vi "Configure Sys (To) Input.vi"(4 "Sys Gate Lev (2.5)":dbl=2.5 format="%.4p", 5 "Sys Trig Lev (2.5)":dbl=2.5 format="%.4p", 6 "Sys Gate Mode":T1(ring), 7 "Sys Trig Edge (T: Rising)":bool=TRUE, 8 "error in (no error)":errorcluster, 9 "Sys Gate Logic (T:High)":bool=TRUE, 10 "Sys Ext Mode":T2(ring), 11 "VISA resource name":refnum<visa-resource-name>) -> (0 "error out":errorcluster, 3 "VISA resource name out":refnum<visa-resource-name>)   [LabVIEW 2013, in "Berkeley Nucleonics 500 Series.lvlib"]
doc: "This VI is used to configure the trigger and gate modes of operation of the main system time (To).\n\nThe parameters \"Trigger Level\", \"Gate Polarity\", \"Trigger Edge\" are only updated when operating in the corresponding mode."
uses:
  Berkeley Nucleonics 500 Series.lvlib
panel:
  # "Trigger"
  # "Simultaneous gating and triggering are currently only supported by the 575."
  # "Gate"
  # "The parameters \"Trigger Level\", \"Gate Polarity\", \"Trigger Edge\" are only updated when operating in the corresponding mode."
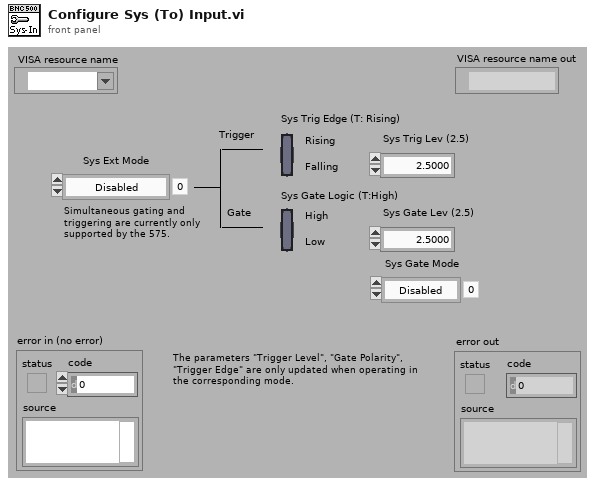
[diagram p1: front panel]
types:
  T1 = enum16{"Disabled", "Pulse Inhibit", "Output Inhibit", "Channel"}
  T2 = enum16{"Disabled", "Triggered", "Gated", "Triggered & Gated"}
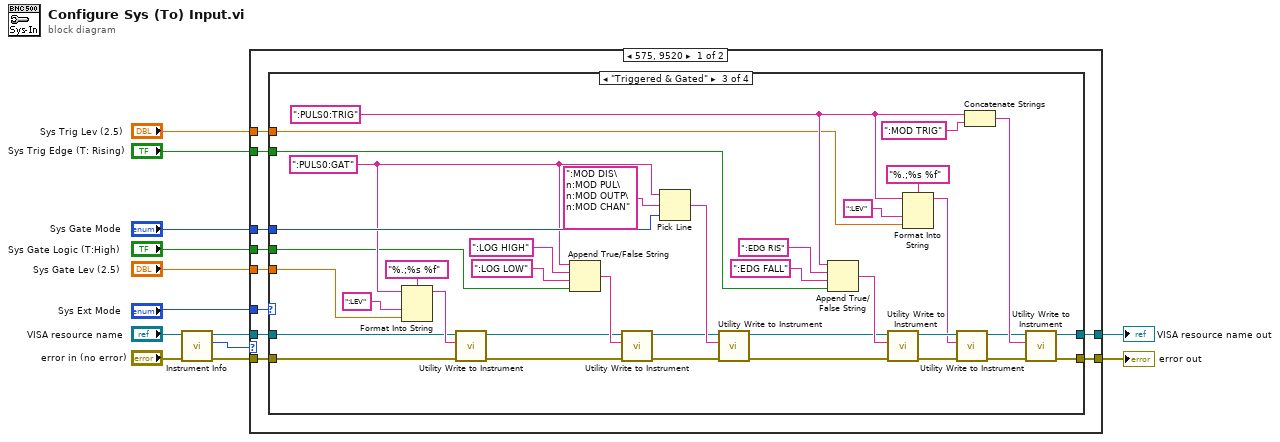
[diagram p0: block diagram]
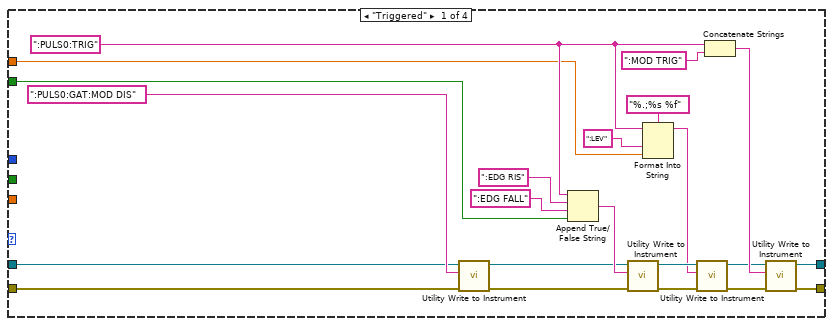
[diagram p2: hidden frame]
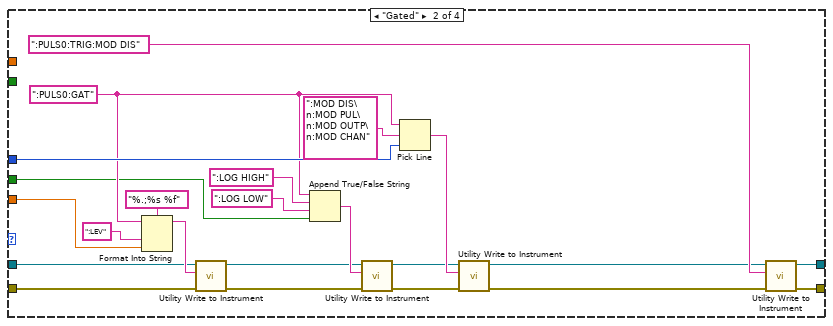
[diagram p3: hidden frame]
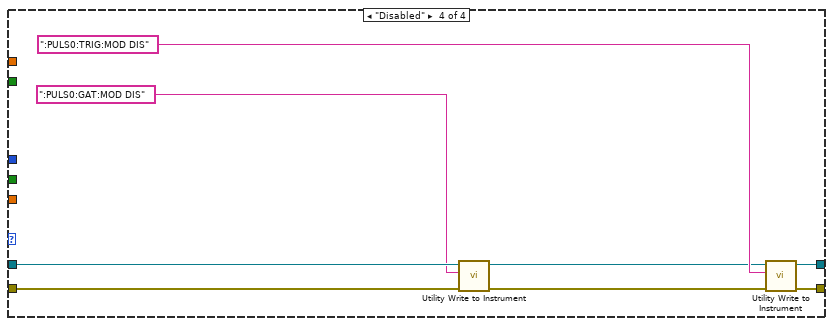
[diagram p4: hidden frame]
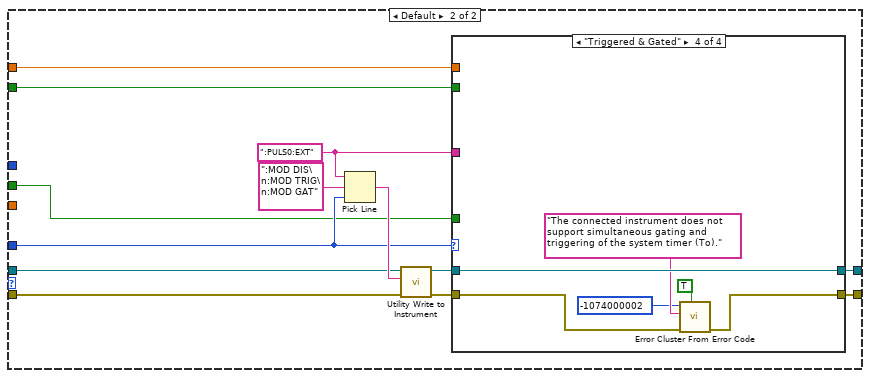
[diagram p5: hidden frame]
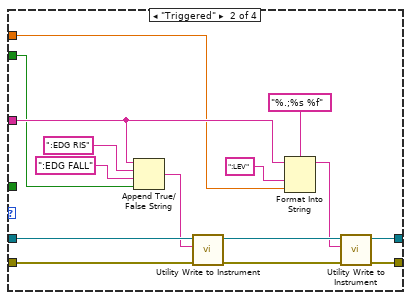
[diagram p7: hidden frame]
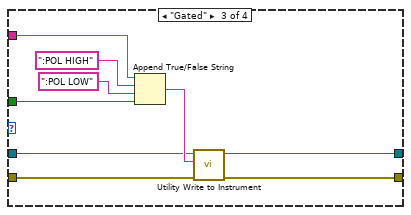
[diagram p8: hidden frame]
diagram:
  n1 = call "Instrument Info.vi"("error in (no error)"="error in (no error)", "VISA resource name"="VISA resource name") -> ("error out"=w8:errorcluster, "Instr Model"=w1:u32, "VISA resource name out"=w7:refnum<visa-resource-name>)  [unwired: 6 in, 1 out]
  n2 = case shown="575, 9520" w1 {
    tunnel: [w23 w121] -> w13
    tunnel: [w22 w120] -> w12
    tunnel: "Sys Ext Mode" -> [w19 w119]
    tunnel: w8 -> [w20 w118]
    tunnel: w7 -> [w21 w117]
    tunnel: "Sys Trig Edge (T: Rising)" -> [w17 w116]
    tunnel: "Sys Trig Lev (2.5)" -> [w18 w115]
    tunnel: "Sys Gate Logic (T:High)" -> [w15 w114]
    tunnel: "Sys Gate Mode" -> [w16 _]
    tunnel: "Sys Gate Lev (2.5)" -> [w14 _]
    frame 575, 9520 {
      n3 = case shown="\"Triggered & Gated\"" w19 {
        tunnel: w21 -> [w25 w54 w76 w108]
        tunnel: w20 -> [w24 w53 w75 w107]
        tunnel: [w41 w65 w99 w112] -> w23
        tunnel: [w42 w66 w100 w113] -> w22
        tunnel: w18 -> [w29 _ w87 _]
        tunnel: w17 -> [w38 _ w96 _]
        tunnel: w16 -> [_ w64 w86 _]
        tunnel: w15 -> [_ w56 w78 _]
        tunnel: w14 -> [_ w55 w77 _]
        frame "Triggered" {
          w30 = ":PULS0:TRIG"
          n4 = call "Utility Write to Instrument.vi"("error in (no error)"=w24, "Write Buffer"=":PULS0:GAT:MOD DIS", "VISA resource name"=w25) -> ("error out"=w27:errorcluster, "VISA resource name out"=w28:refnum<visa-resource-name>)  [unwired: 6 in, 1 out]
          n5 = Append True/False String(1:w38, 2:":EDG FALL", 3:":EDG RIS", 4:w30) -> (0:w43:string)
          n6 = call "Utility Write to Instrument.vi"("error in (no error)"=w27, "Write Buffer"=w43, "VISA resource name"=w28) -> ("error out"=w33:errorcluster, "VISA resource name out"=w32:refnum<visa-resource-name>)  [unwired: 6 in, 1 out]
          n7 = Format Into String(format string="%.;%s %f", initial string=w30, ":LEV", w29) -> (resulting string=w31:string)  [unwired: 1 in, 1 out]
          n8 = call "Utility Write to Instrument.vi"("error in (no error)"=w33, "Write Buffer"=w31, "VISA resource name"=w32) -> ("error out"=w35:errorcluster, "VISA resource name out"=w34:refnum<visa-resource-name>)  [unwired: 6 in, 1 out]
          n9 = Concatenate Strings(w30, ":MOD TRIG") -> (w39:string)
          n10 = call "Utility Write to Instrument.vi"("error in (no error)"=w35, "Write Buffer"=w39, "VISA resource name"=w34) -> ("error out"=w42:errorcluster, "VISA resource name out"=w41:refnum<visa-resource-name>)  [unwired: 6 in, 1 out]
        }
        frame "Gated" {
          w57 = ":PULS0:GAT"
          n11 = Format Into String(format string="%.;%s %f", initial string=w57, ":LEV", w55) -> (resulting string=w63:string)  [unwired: 1 in, 1 out]
          n12 = call "Utility Write to Instrument.vi"("error in (no error)"=w53, "Write Buffer"=w63, "VISA resource name"=w54) -> ("error out"=w52:errorcluster, "VISA resource name out"=w51:refnum<visa-resource-name>)  [unwired: 6 in, 1 out]
          n13 = Append True/False String(1:w56, 2:":LOG LOW", 3:":LOG HIGH", 4:w57) -> (0:w60:string)
          n14 = call "Utility Write to Instrument.vi"("error in (no error)"=w52, "Write Buffer"=w60, "VISA resource name"=w51) -> ("error out"=w50:errorcluster, "VISA resource name out"=w49:refnum<visa-resource-name>)  [unwired: 6 in, 1 out]
          n15 = Pick Line(string ("")=w57, multi-line string=":MOD DIS\n:MOD PUL\n:MOD OUTP\n:MOD CHAN", line index=w64) -> (output string=w68:string)
          n16 = call "Utility Write to Instrument.vi"("error in (no error)"=w50, "Write Buffer"=w68, "VISA resource name"=w49) -> ("error out"=w47:errorcluster, "VISA resource name out"=w46:refnum<visa-resource-name>)  [unwired: 6 in, 1 out]
          n17 = call "Utility Write to Instrument.vi"("error in (no error)"=w47, "Write Buffer"=":PULS0:TRIG:MOD DIS", "VISA resource name"=w46) -> ("error out"=w66:errorcluster, "VISA resource name out"=w65:refnum<visa-resource-name>)  [unwired: 6 in, 1 out]
        }
        frame "Triggered & Gated" {
          w79 = ":PULS0:GAT"
          w88 = ":PULS0:TRIG"
          n18 = Format Into String(format string="%.;%s %f", initial string=w79, ":LEV", w77) -> (resulting string=w85:string)  [unwired: 1 in, 1 out]
          n19 = call "Utility Write to Instrument.vi"("error in (no error)"=w75, "Write Buffer"=w85, "VISA resource name"=w76) -> ("error out"=w74:errorcluster, "VISA resource name out"=w73:refnum<visa-resource-name>)  [unwired: 6 in, 1 out]
          n20 = Append True/False String(1:w78, 2:":LOG LOW", 3:":LOG HIGH", 4:w79) -> (0:w82:string)
          n21 = call "Utility Write to Instrument.vi"("error in (no error)"=w74, "Write Buffer"=w82, "VISA resource name"=w73) -> ("error out"=w72:errorcluster, "VISA resource name out"=w71:refnum<visa-resource-name>)  [unwired: 6 in, 1 out]
          n22 = Pick Line(string ("")=w79, multi-line string=":MOD DIS\n:MOD PUL\n:MOD OUTP\n:MOD CHAN", line index=w86) -> (output string=w102:string)
          n23 = call "Utility Write to Instrument.vi"("error in (no error)"=w72, "Write Buffer"=w102, "VISA resource name"=w71) -> ("error out"=w69:errorcluster, "VISA resource name out"=w70:refnum<visa-resource-name>)  [unwired: 6 in, 1 out]
          n24 = Append True/False String(1:w96, 2:":EDG FALL", 3:":EDG RIS", 4:w88) -> (0:w103:string)
          n25 = call "Utility Write to Instrument.vi"("error in (no error)"=w69, "Write Buffer"=w103, "VISA resource name"=w70) -> ("error out"=w91:errorcluster, "VISA resource name out"=w90:refnum<visa-resource-name>)  [unwired: 6 in, 1 out]
          n26 = Format Into String(format string="%.;%s %f", initial string=w88, ":LEV", w87) -> (resulting string=w89:string)  [unwired: 1 in, 1 out]
          n27 = call "Utility Write to Instrument.vi"("error in (no error)"=w91, "Write Buffer"=w89, "VISA resource name"=w90) -> ("error out"=w93:errorcluster, "VISA resource name out"=w92:refnum<visa-resource-name>)  [unwired: 6 in, 1 out]
          n28 = Concatenate Strings(w88, ":MOD TRIG") -> (w97:string)
          n29 = call "Utility Write to Instrument.vi"("error in (no error)"=w93, "Write Buffer"=w97, "VISA resource name"=w92) -> ("error out"=w100:errorcluster, "VISA resource name out"=w99:refnum<visa-resource-name>)  [unwired: 6 in, 1 out]
        }
        frame "Disabled" {
          n30 = call "Utility Write to Instrument.vi"("error in (no error)"=w107, "Write Buffer"=":PULS0:GAT:MOD DIS", "VISA resource name"=w108) -> ("error out"=w109:errorcluster, "VISA resource name out"=w110:refnum<visa-resource-name>)  [unwired: 6 in, 1 out]
          n31 = call "Utility Write to Instrument.vi"("error in (no error)"=w109, "Write Buffer"=":PULS0:TRIG:MOD DIS", "VISA resource name"=w110) -> ("error out"=w113:errorcluster, "VISA resource name out"=w112:refnum<visa-resource-name>)  [unwired: 6 in, 1 out]
        }
      }
    }
    frame Default {
      w125 = ":PULS0:EXT"
      n32 = Pick Line(string ("")=w125, multi-line string=":MOD DIS\n:MOD TRIG\n:MOD GAT", line index=w119) -> (output string=w126:string)
      n33 = call "Utility Write to Instrument.vi"("error in (no error)"=w118, "Write Buffer"=w126, "VISA resource name"=w117) -> ("error out"=w122:errorcluster, "VISA resource name out"=w123:refnum<visa-resource-name>)  [unwired: 6 in, 1 out]
      n34 = case shown="\"Triggered & Gated\"" w119 {
        tunnel: w125 -> [_ w134 w152 _]
        tunnel: w123 -> [w128 w141 w146 w158]
        tunnel: w122 -> [w127 w140 w145 w153]
        tunnel: [w128 w132 w148 w158] -> w121
        tunnel: [w127 w131 w147 w154] -> w120
        tunnel: w116 -> [_ w130 _ _]
        tunnel: w115 -> [_ w129 _ _]
        tunnel: w114 -> [_ _ w144 _]
        frame "Disabled" {
        }
        frame "Triggered" {
          n35 = Append True/False String(1:w130, 2:":EDG FALL", 3:":EDG RIS", 4:w134) -> (0:w139:string)
          n36 = call "Utility Write to Instrument.vi"("error in (no error)"=w140, "Write Buffer"=w139, "VISA resource name"=w141) -> ("error out"=w137:errorcluster, "VISA resource name out"=w138:refnum<visa-resource-name>)  [unwired: 6 in, 1 out]
          n37 = Format Into String(format string="%.;%s %f", initial string=w134, ":LEV", w129) -> (resulting string=w133:string)  [unwired: 1 in, 1 out]
          n38 = call "Utility Write to Instrument.vi"("error in (no error)"=w137, "Write Buffer"=w133, "VISA resource name"=w138) -> ("error out"=w131:errorcluster, "VISA resource name out"=w132:refnum<visa-resource-name>)  [unwired: 6 in, 1 out]
        }
        frame "Gated" {
          n39 = Append True/False String(1:w144, 2:":POL LOW", 3:":POL HIGH", 4:w152) -> (0:w149:string)
          n40 = call "Utility Write to Instrument.vi"("error in (no error)"=w145, "Write Buffer"=w149, "VISA resource name"=w146) -> ("error out"=w147:errorcluster, "VISA resource name out"=w148:refnum<visa-resource-name>)  [unwired: 6 in, 1 out]
        }
        frame "Triggered & Gated" {
          n41 = call <vilib>:"Error Cluster From Error Code.vi"("show call chain? (False)"=TRUE, "error in (no error)"=w153, "error message (\"\")"="The connected instrument does not support simultaneous gating and triggering of the system timer (To)." ("Source (VI Name)"), "error code (0)"=-1074000002 ("Code")) -> ("error out"=w154:errorcluster)  [unwired: 5 in]
        }
      }
    }
  }
  "error out" <- w12
  "VISA resource name out" <- w13
